vi "Update Tipstrip.vi"(8 "error in (no error)":errorcluster, 10 "Assert Message":T1, 11 "Main Display in":refnum<class "Main Display.lvclass">) -> (0 "error out":errorcluster, 3 "Main Display out":refnum<class "Main Display.lvclass">)   [LabVIEW 2016]
doc: "Updates the tip strip for the specified control reference with a new string"
uses:
  Assert Display/Assert Display.lvlib
  <resource>/AFDebug/AF Debug.lvlib
  Main Display.lvclass
  D:/Work/Projects/Actor_Assert_API/Base UI Component/Base UI Component/Base UI Component.lvclass
  D:/Work/Projects/Actor_Assert_API/Base UI Actor/Base UI Actor/Base UI Actor.lvclass
  C:/Program Files (x86)/National Instruments/LabVIEW 2016/vi.lib/ActorFramework/Actor/Actor.lvclass
  Assert API Components/VI References.ctl
  Assert API Components/Assert API Components.lvlib
  Assert API Components/Message Data.ctl
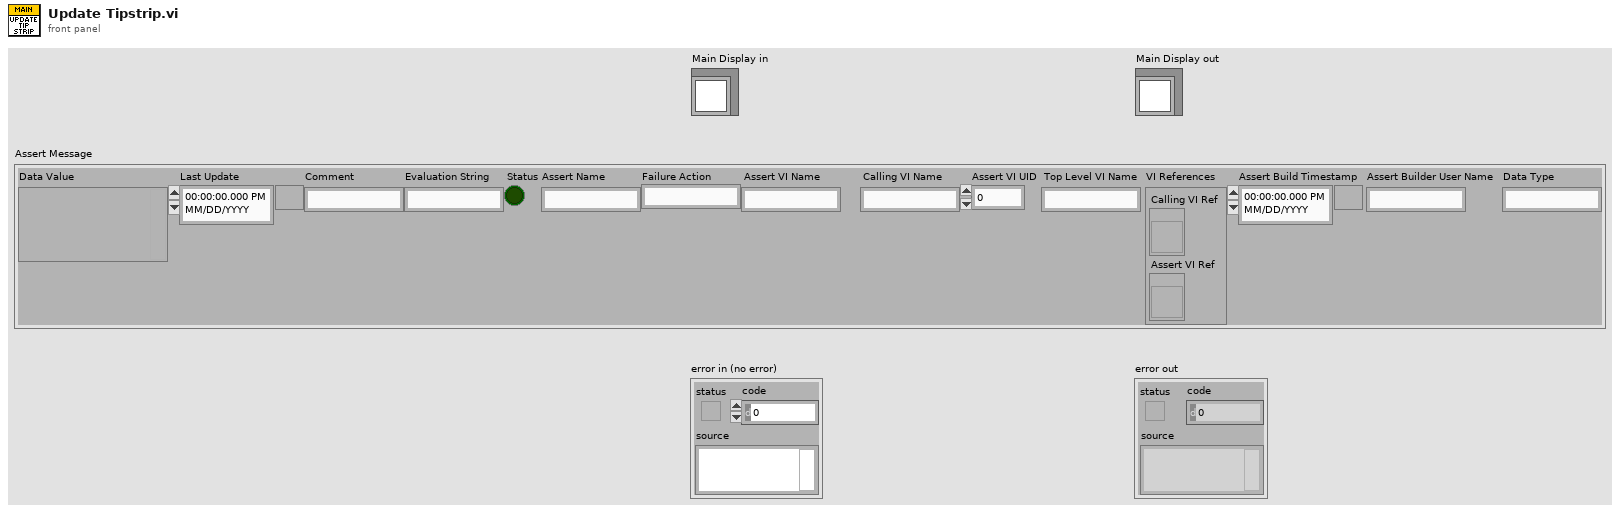
[diagram p1: front panel]
types:
  T1 = typedef "Assert API Components.lvlib/Message Data.ctl" = cluster{"Data Value":variant, "Last Update":timestamp, "Comment":string, "Evaluation String":string, "Status":bool, "Assert Name":string, "Failure Action":string, "Assert VI Name":string, "Calling VI Name":string, "Assert VI UID":i32, "Top Level VI Name":string, "VI References":T2, "Assert Build Timestamp":timestamp, "Assert Builder User Name":string, "Data Type":string}
  T2 = typedef "Assert API Components.lvlib/VI References.ctl" = cluster{"Calling VI Ref":refnum<vi>, "Assert VI Ref":refnum<vi>}
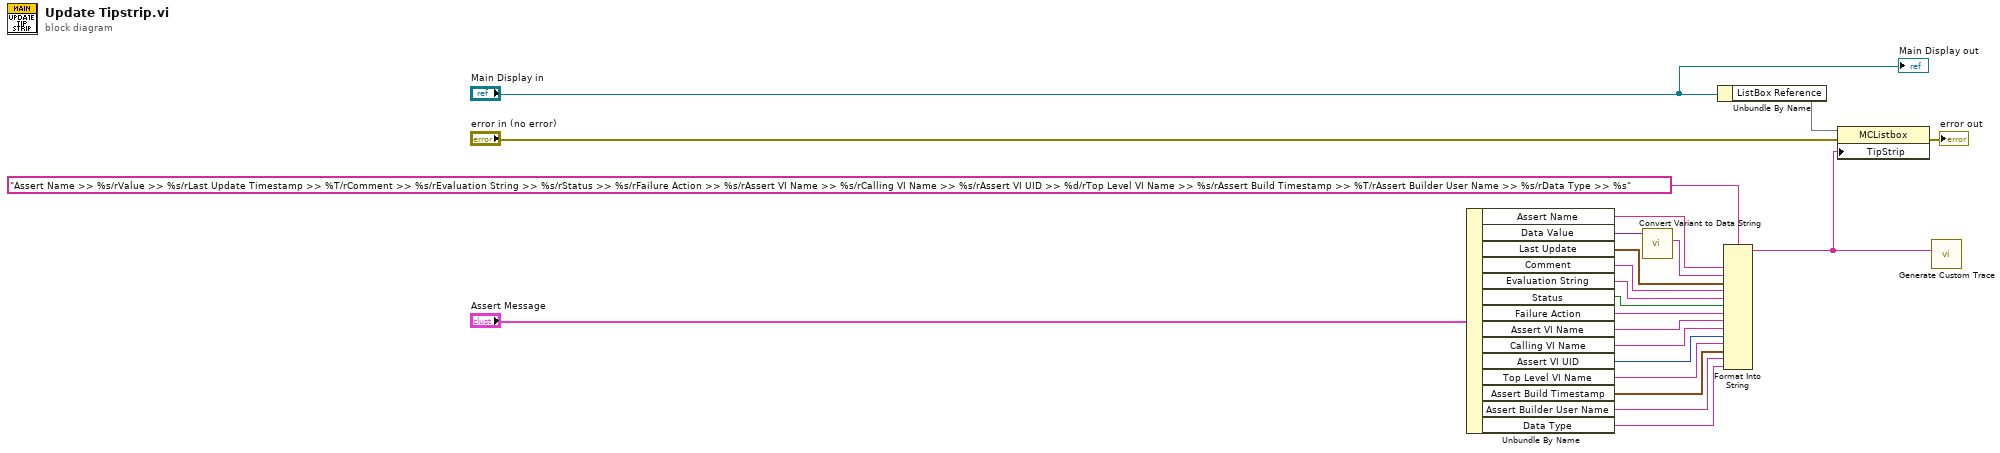
[diagram p0: block diagram]
diagram:
  n1 = Unbundle By Name("Assert Message") -> ("Assert Name"=w16:string, "Data Value"=w17:variant, "Last Update"=w14:timestamp, "Comment"=w13:string, "Evaluation String"=w12:string, "Status"=w11:bool, "Failure Action"=w10:string, "Assert VI Name"=w9:string, "Calling VI Name"=w8:string, "Assert VI UID"=w7:i32, "Top Level VI Name"=w6:string, "Assert Build Timestamp"=w5:timestamp, "Assert Builder User Name"=w4:string, "Data Type"=w3:string)
  n2 = call "Convert Variant to Data String.vi"("Data Value"=w17) -> ("Data Value String"=w15:string)  [unwired: 9 in, 1 out]
  n3 = Unbundle By Name("Main Display in") -> ("ListBox Reference"=w20)
  n4 = Format Into String(format string="Assert Name >> %s/rValue >> %s/rLast Update Timestamp >> %T/rComment >> %s/rEvaluation String >> %s/rStatus >> %s/rFailure Action >> %s/rAssert VI Name >> %s/rCalling VI Name >> %s/rAssert VI UID >> %d/rTop Level VI Name >> %s/rAssert Build Timestamp >> %T/rAssert Builder User Name >> %s/rData Type >> %s", w16, w15, w14, w13, w12, w11, w10, w9, w8, w7, w6, w5, w4, w3) -> (resulting string=w1:string)  [unwired: 2 in, 1 out]
  n5 = property class="MCListbox"(reference=w20, error in="error in (no error)", "TipStrip"=w1) -> (error out=→"error out":errorcluster)  [unwired: 1 out]
  n6 = call <resource>:"Generate Custom Trace.vi"("Custom Action"=w1) -> ()  [unwired: 11 in]
  "Main Display out" <- "Main Display in"
